vi "Table Pick Row Border V2.vi"(6 "# header rows":i32, 7 "Data Row Back Ground color":T10={"color"=16777225, "at each"=0}, 8 "columnWidth (points)":sgl[](array[numeric]), 9 "Row format with ref [ ]":T9(array[cluster]), 10 "i":i32, 11 "N":i32) -> (0 "columnWidth (points) out":sgl[](array[numeric]), 1 "Row format with ref":T8, 3 "Background Color":u32(colorbox))   [LabVIEW 2019, in "Exaprom PDF.lvlib"]
doc: "Version 1.0\nDeveloped by Jean-Marc Simard\nCopyright © 2010, Exaprom Inc.\nAll rights reserved.\nLicense: BSD"
uses:
  Controls/Table Controls/Row Back Ground color Datas.ctl
  Controls/Table Controls/Table Custom type Titles or Datas.ctl
  C:/work/niobrara_lv/labview pdf writer fixing/DLL/itextsharp.dll
  DLL/itextsharp.dll
  Controls/Font Controls/Font size.ctl
  Controls/Text Controls/Texte alignement.ctl
  Controls/Table Controls/Cell Vertical alignment.ctl
  Controls/Text Controls/Unicode/ASCII or Unicode.ctl
  Controls/Text Controls/Unicode/Character type.ctl
  Controls/Text Controls/Unicode/Writing direction.ctl
  General/Stop if it True.vi
  Exaprom PDF.lvlib
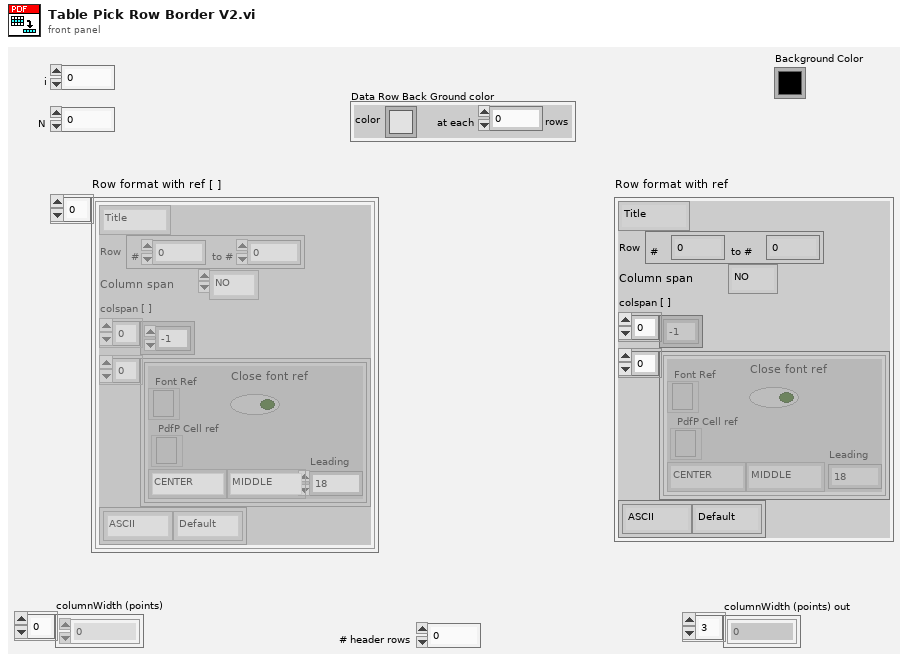
[diagram p1: front panel]
types:
  T1 = typedef "Exaprom PDF.lvlib/Table Custom type Titles or Datas.ctl" = enum16{"Title", "Data"}
  T2 = typedef "Exaprom PDF.lvlib/Font size.ctl" = sgl
  T3 = typedef "Exaprom PDF.lvlib/Texte alignement.ctl" = enum16{"Select", "CENTER", "JUSTIFY", "LEFT", "RIGHT"}
  T4 = typedef "Exaprom PDF.lvlib/Cell Vertical alignment.ctl" = enum16{"TOP", "MIDDLE", "BOTTOM"}
  T5 = typedef "Exaprom PDF.lvlib/ASCII or Unicode.ctl" = cluster{"Type":T6, "Direction":T7}
  T6 = typedef "Exaprom PDF.lvlib/Character type.ctl" = enum16{"ASCII", "Unicode"}
  T7 = typedef "Exaprom PDF.lvlib/Writing direction.ctl" = enum16{"Default", "NO BIDI", "LTR", "RTL"}
  T8 = cluster{"Titles or datas":T1, "Row":cluster{"#":i16, "to #":i16}, "Column span":enum16{"NO", "YES"}, "colspan [ ]":i8[], "Cell [ ]":cluster{"Font Ref":refnum<k24>, "Leading":T2, "PdfP Cell ref":refnum<k24>, "Horizontal":T3, "Vertical":T4, "Close font ref":bool}[], "ASCII or Unicode":T5}
  T9 = cluster{"Titles or datas":T1, "Row":cluster{"#":i16, "to #":i16}, "Column span":enum16{"NO", "YES"}, "colspan [ ]":i8[], "Cell [ ]":cluster{"Font Ref":refnum<k24>, "Leading":T2, "PdfP Cell ref":refnum<k24>, "Horizontal":T3, "Vertical":T4, "Close font ref":bool}[], "ASCII or Unicode":T5}[]
  T10 = typedef "Exaprom PDF.lvlib/Row Back Ground color Datas.ctl" = cluster{"color":u32, "at each":i16}
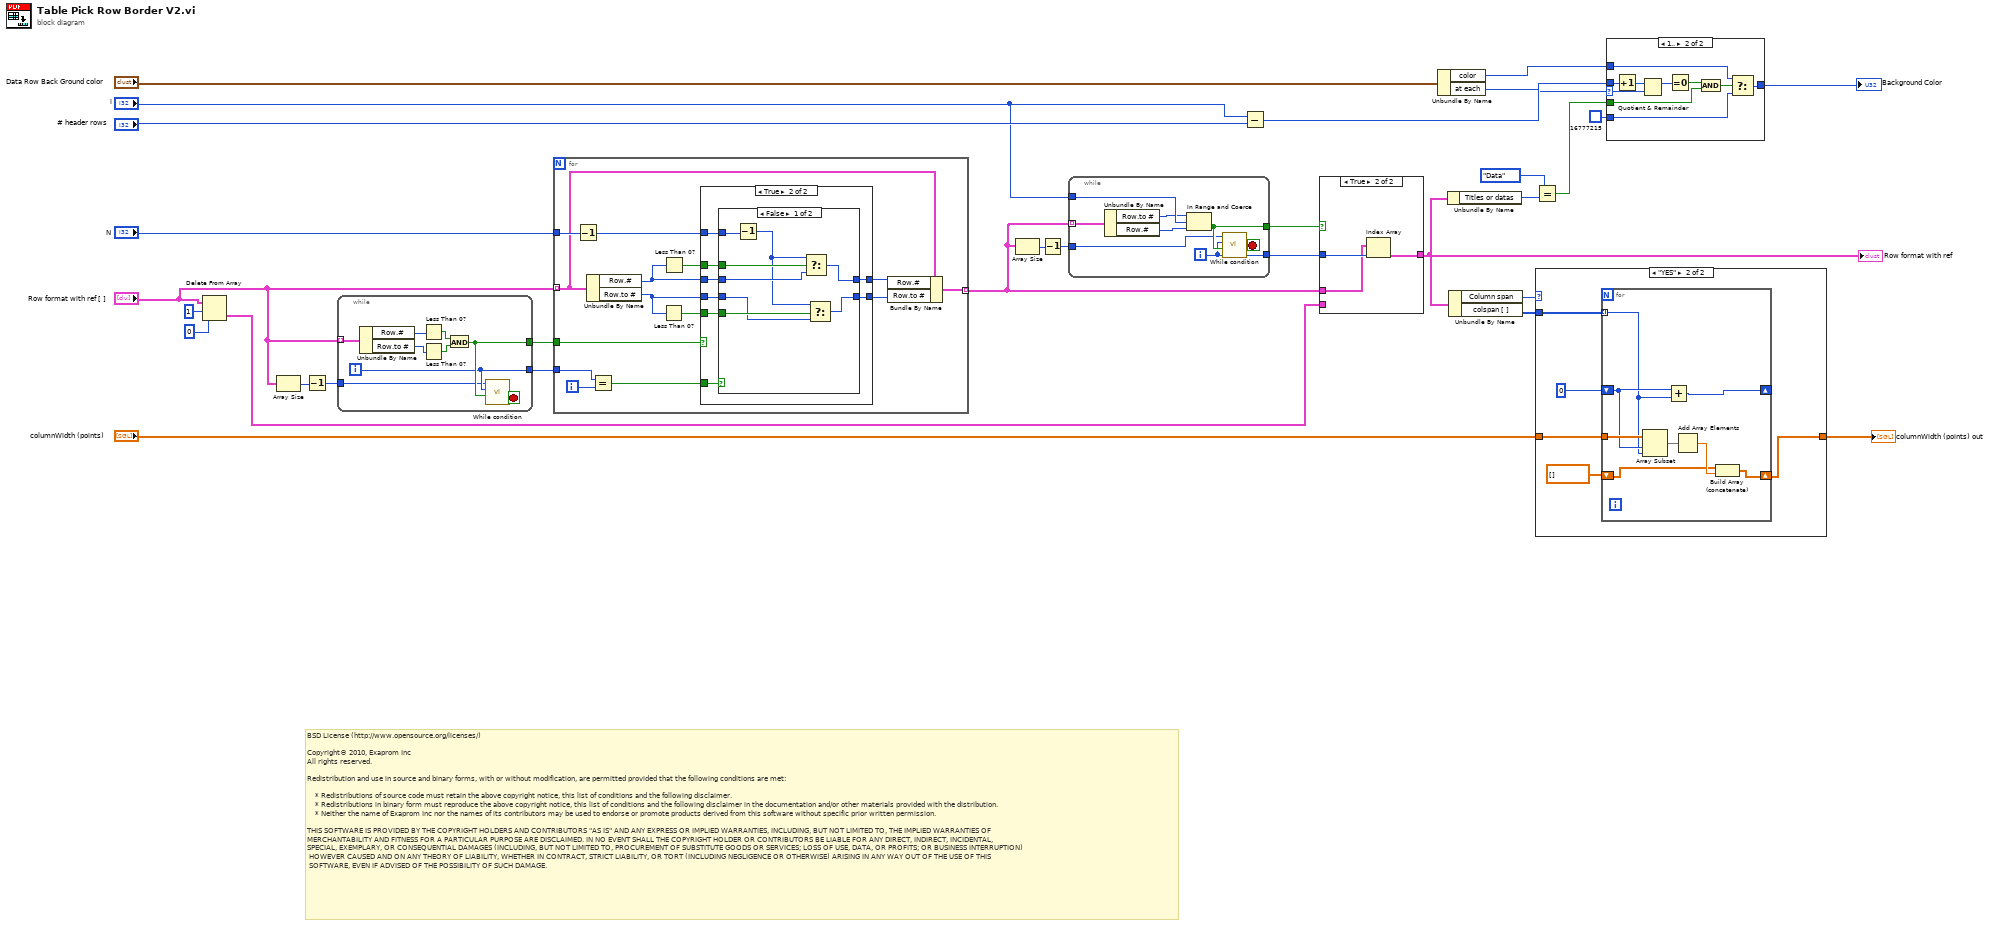
[diagram p0: block diagram]
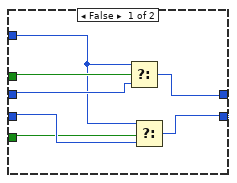
[diagram p4: hidden frame]
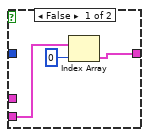
[diagram p6: hidden frame]
diagram:
  # "BSD License (http://www.opensource.org/licenses/)\n\nCopyright© 2010, Exaprom Inc\nAll rights reserved.\n\nRedistribution and use in source and binary forms, with or without modification, are permitted provided that the following conditions are met:\n\n    * Redistributions of source code must retain the above copyright notice, this list of conditions and the following disclaimer.\n    * Redistributions in binary form must reproduce the above copyright notice, this list of conditions and the following disclaimer in the documentation and/or other materials provided with the distribution.\n    * Neither the name of Exaprom Inc nor the names of its contributors may be used to endorse or promote products derived from this software without specific prior written permission.\n\nTHIS SOFTWARE IS PROVIDED BY THE COPYRIGHT HOLDERS AND CONTRIBUTORS \"AS IS\" AND ANY EXPRESS OR IMPLIED WARRANTIES, INCLUDING, BUT NOT LIMITED TO, THE IMPLIED WARRANTIES OF \nMERCHANTABILITY AND FITNESS FOR A PARTICULAR PURPOSE ARE DISCLAIMED. IN NO EVENT SHALL THE COPYRIGHT HOLDER OR CONTRIBUTORS BE LIABLE FOR ANY DIRECT, INDIRECT, INCIDENTAL,\nSPECIAL, EXEMPLARY, OR CONSEQUENTIAL DAMAGES (INCLUDING, BUT NOT LIMITED TO, PROCUREMENT OF SUBSTITUTE GOODS OR SERVICES; LOSS OF USE, DATA, OR PROFITS; OR BUSINESS INTERRUPTION)\n HOWEVER CAUSED AND ON ANY THEORY OF LIABILITY, WHETHER IN CONTRACT, STRICT LIABILITY, OR TORT (INCLUDING NEGLIGENCE OR OTHERWISE) ARISING IN ANY WAY OUT OF THE USE OF THIS\n SOFTWARE, EVEN IF ADVISED OF THE POSSIBILITY OF SUCH DAMAGE."
  n1 = Delete From Array(array="Row format with ref [ ]", length=1, index=0) -> (deleted portion=w21:T9)  [unwired: 1 out]
  n2 = Array Size(array="Row format with ref [ ]") -> (size(s)=w19:i32)
  n3 = Decrement(x=w19) -> (x-1=w20:i32)
  n4 = while {
    tunnel: "Row format with ref [ ]" -> [w39] mode=indexing
    tunnel: [w33] -> w28
    tunnel: [w32] -> w27
    tunnel: w20 -> [w31]
    i -> [w32]
    stop <- w34 stop-if-true
    n5 = Unbundle By Name(w39) -> ("Row.#"=w38:i16, "Row.to #"=w37:i16)
    n6 = Less Than 0?(x=w38) -> (x < 0?=w35:bool)
    n7 = Less Than 0?(x=w37) -> (x < 0?=w36:bool)
    n8 = And(x=w35, y=w36) -> (x .and. y?=w33:bool)
    n9 = call-poly "While condition.vi"("Test"=w33, "i"=w32, "N"=w31) -> ("Action"=w34:bool)  [unwired: 5 out]
  }
  n10 = for {
    tunnel: "Row format with ref [ ]" -> [w45] mode=indexing
    tunnel: w28 -> [w53]
    tunnel: w27 -> [w51]
    tunnel: "N" -> [w47]
    tunnel: [w40] -> w16 mode=indexing
    i -> [w52]
    n11 = Decrement(x=w47) -> (x-1=w46:i32)
    n12 = Unbundle By Name(w45) -> ("Row.#"=w49:i16, "Row.to #"=w48:i16)
    n13 = Equal?(x=w51, y=w52) -> (x = y?=w50:bool)
    n14 = Less Than 0?(x=w48) -> (x < 0?=w42:bool)
    n15 = Less Than 0?(x=w49) -> (x < 0?=w41:bool)
    n16 = case shown="True" w53 {
      tunnel: w50 -> [_ w68]
      tunnel: w49 -> [w60 w67]
      tunnel: w48 -> [w58 w66]
      tunnel: w46 -> [w54 w65]
      tunnel: [w55 w64] -> w44
      tunnel: [w56 w63] -> w43
      tunnel: w42 -> [w57 w62]
      tunnel: w41 -> [w59 w61]
      frame False {
        n17 = Select(t=w54, s=w59, f=w60) -> (s? t:f=w55:i32)
        n18 = Select(t=w54, s=w57, f=w58) -> (s? t:f=w56:i32)
      }
      frame True {
        n19 = case shown="False" w68 {
          tunnel: w67 -> [w74 _]
          tunnel: w66 -> [w70 _]
          tunnel: [w73 w77] -> w64
          tunnel: [w69 w77] -> w63
          tunnel: w65 -> [w76 w77]
          tunnel: w62 -> [w72 _]
          tunnel: w61 -> [w75 _]
          frame False {
            n20 = Decrement(x=w76) -> (x-1=w71:i32)
            n21 = Select(t=w71, s=w75, f=w74) -> (s? t:f=w73:i32)
            n22 = Select(t=w71, s=w72, f=w70) -> (s? t:f=w69:i32)
          }
          frame True {
          }
        }
      }
    }
    n23 = Bundle By Name(cluster=w45, "Row.#"=w44, "Row.to #"=w43) -> (w40:T8)
  }
  n24 = Array Size(array=w16) -> (size(s)=w18:i32)
  n25 = Decrement(x=w18) -> (x-1=w17:i32)
  n26 = while {
    tunnel: w16 -> [w85] mode=indexing
    tunnel: "i" -> [w84]
    tunnel: [w79] -> w29
    tunnel: [w80] -> w30
    tunnel: w17 -> [w78]
    i -> [w79]
    stop <- w81 stop-if-true
    n27 = Unbundle By Name(w85) -> ("Row.to #"=w82:i16, "Row.#"=w83:i16)
    n28 = In Range and Coerce(upper limit=w82, x=w84, lower limit=w83) -> (In Range?=w80:bool)  [unwired: 1 out]
    n29 = call-poly "While condition.vi"("Test"=w80, "i"=w79, "N"=w78) -> ("Action"=w81:bool)  [unwired: 5 out]
  }
  n30 = Subtract(x="i", y="# header rows") -> (x-y=w3:i32)
  n31 = case shown="True" w30 {
    tunnel: w29 -> [_ w91]
    tunnel: w21 -> [w88 _]
    tunnel: [w86 w90] -> w10
    tunnel: w16 -> [_ w89]
    frame False {
      n32 = Index Array(array=w88, index=0) -> (element=w86:T8)
    }
    frame True {
      n33 = Index Array(array=w89, index=w91) -> (element=w90:T8)
    }
  }
  "Row format with ref" <- w10
  n34 = Unbundle By Name("Data Row Back Ground color") -> ("color"=w25:u32, "at each"=w2:i16)
  n35 = Unbundle By Name(w10) -> ("Titles or datas"=w13:T1)
  n36 = Unbundle By Name(w10) -> ("Column span"=w9:enum16{"NO", "YES"}, "colspan [ ]"=w7:i8[])
  n37 = Equal?(x=Table_Custom_type_Titles_or_Datas."Data", y=w13) -> (x = y?=w11:bool)
  n38 = case shown="\"YES\"" w9 {
    tunnel: "columnWidth (points)" -> [w92 w94]
    tunnel: [w92 w93] -> w6
    tunnel: w7 -> [_ w97]
    frame "NO", Default {
    }
    frame "YES" {
      n39 = for {
        tunnel: w97 -> [w103] mode=indexing
        shift-right: [w98] -> _
        shift-left: i8 0 ("span") -> [w104]
        shift-right: [w99] -> w93
        shift-left: sgl[] [] ("columnWidth (points)") -> [w100]
        tunnel: w94 -> [w105]
        n40 = Array Subset(array=w105, index=w104, length=w103) -> (w102:sgl[])
        n41 = Add(x=w104, y=w103) -> (x+y=w98:i8)
        n42 = Add Array Elements(numeric array=w102) -> (sum=w101:sgl)
        n43 = Build Array (concatenate)(w100, w101) -> (w99:sgl[])
      }
    }
  }
  "columnWidth (points) out" <- w6
  n44 = case shown="1.." w2 {
    selector: w2 -> [_ w107]
    tunnel: w25 -> [_ w114]
    tunnel: u32 16777215 ("Color") -> [w106 w113]
    tunnel: [w106 w112] -> w23
    tunnel: w11 -> [_ w110]
    tunnel: w3 -> [_ w108]
    frame 0, Default {
    }
    frame 1.. {
      n45 = Increment(x=w108) -> (x+1=w116:i32)
      n46 = Quotient & Remainder(x=w116, y=w107) -> (x-y*floor(x/y)=w115:i32)  [unwired: 1 out]
      n47 = Equal To 0?(x=w115) -> (x = 0?=w111:bool)
      n48 = And(x=w111, y=w110) -> (x .and. y?=w109:bool)
      n49 = Select(t=w114, s=w109, f=w113) -> (s? t:f=w112:u32)
    }
  }
  "Background Color" <- w23
